vi "Close.vi"(7 "Delay":u32=10 format="%.0fms", 8 "error in (no error)":errorcluster, 10 "Clean up":bool=TRUE, 11 "File in":refnum<class "File.lvclass">) -> (0 "error out":errorcluster, 1 "Actually closed":bool, 2 "File Path":path, 3 "File out":refnum<class "File.lvclass">)   [LabVIEW 2019, in "File.lvclass"]
uses:
  File.lvclass
  File.lvclass/File.ctl
  Read Is open.vi
  Read tdms stream.vi
  Write tdms stream.vi
  Write Is open.vi
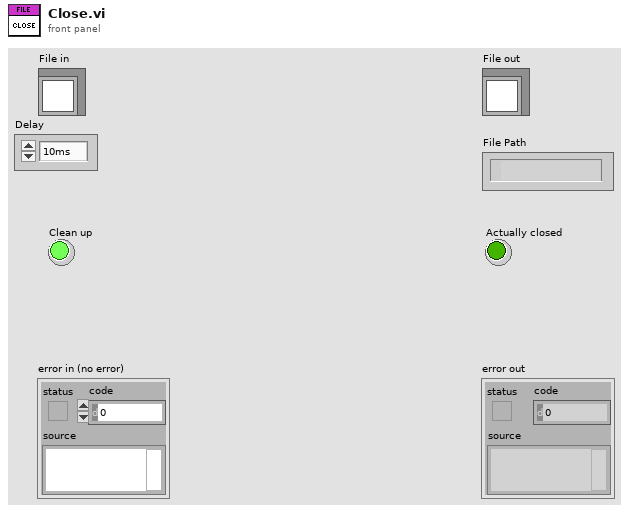
[diagram p1: front panel]
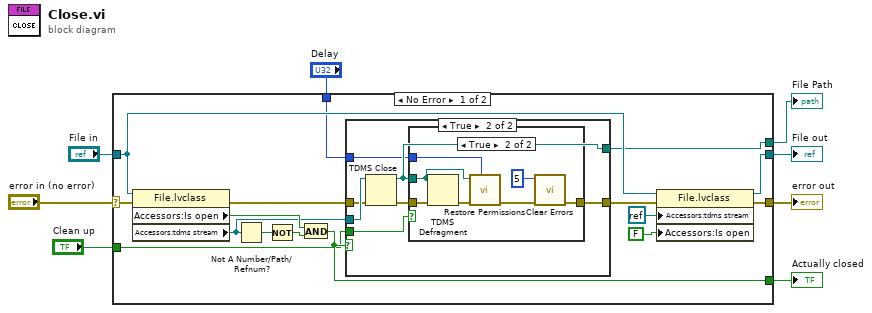
[diagram p0: block diagram]
diagram:
  n1 = case shown="No Error" "error in (no error)" {
    selector: "error in (no error)" -> [w19 w42]
    tunnel: [w13 w42] -> w7
    tunnel: [w17 w41] -> w5
    tunnel: "File in" -> [w18 w41]
    tunnel: [w12 _] -> w4
    tunnel: [w11 _] -> w3
    tunnel: "Clean up" -> [w10 _]
    tunnel: "Delay" -> [w9 _]
    frame No Error {
      n2 = property class="File.lvclass"(reference=w18, error in=w19) -> (error out=w24:errorcluster, "Accessors:Is open"=w23:bool, "Accessors:tdms stream"=w22:refnum<k34>)  [unwired: 1 out]
      n3 = Not A Number/Path/Refnum?(number/path/refnum=w22) -> (NaN/Path/Refnum?=w21:bool)
      n4 = Not(x=w21) -> (.not. x?=w20:bool)
      n5 = And(x=w23, y=w20) -> (x .and. y?=w12:bool)
      n6 = case shown="True" w12 {
        tunnel: w24 -> [w25 w31]
        tunnel: w22 -> [_ w32]
        tunnel: [w25 w27] -> w14
        tunnel: [_ w29] -> w11
        tunnel: w10 -> [_ w30]
        tunnel: w9 -> [_ w26]
        frame False {
        }
        frame True {
          n7 = TDMS Close(8:w31, 11:w32) -> (0:w28:errorcluster, 3:w29:path)
          n8 = case shown="True" w30 {
            tunnel: w29 -> [_ w35]
            tunnel: w28 -> [w33 w37]
            tunnel: [w33 w36] -> w27
            tunnel: w26 -> [_ w34]
            frame False {
            }
            frame True {
              n9 = TDMS Defragment(4:w37, 7:w35) -> (0:w38:errorcluster)
              n10 = call "Restore Permissions.vi"("Delay"=w34, "Error In"=w38, "File Path"=w35) -> ("Error Out"=w40:errorcluster)  [unwired: 5 in, 3 out]
              n11 = call <vilib>:"Clear Errors.vi"("error in (no error)"=w40, "specific error code to clear (0: all)"=5) -> ("error out"=w36:errorcluster)  [unwired: 4 in, 1 out]
            }
          }
        }
      }
      n12 = property class="File.lvclass"(reference=w18, error in=w14, "Accessors:tdms stream"=refnum<k0> refnum, "Accessors:Is open"=FALSE ("Is open")) -> (reference out=w17:refnum<class "File.lvclass">, error out=w13:errorcluster)
    }
    frame Error {
    }
  }
  "error out" <- w7
  "File out" <- w5
  "Actually closed" <- w4
  "File Path" <- w3
